vi "Open Handle2.vi"(0 "server address":string caption="サーバアドレス", 5 "from":string caption="送信者", 7 "username":string caption="ユーザ名", 9 "password":string caption="パスワード", 11 "error in (no error)":errorcluster caption="エラー入力（エラーなし）", 12 "use TLS (false)":bool caption="TLSを使用 (FALSE)") -> (4 "handles cluster out":T1 caption="ハンドルクラスター出力", 15 "error out":errorcluster caption="エラー出力")   [LabVIEW 2015]
doc: "指定されたSMTPサーバを使用して新しいハンドルクラスターを作成します。作成したハンドルは、「Close Handle2」VIを使用して閉じる必要があります。"
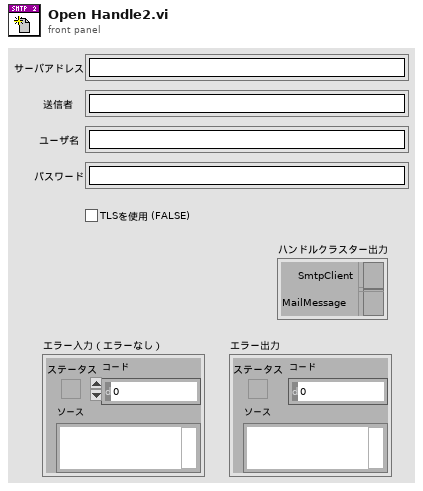
[diagram p1: front panel]
types:
  T1 = cluster{"SmtpClient":refnum<k24>, "MailMessage":refnum<k24>}
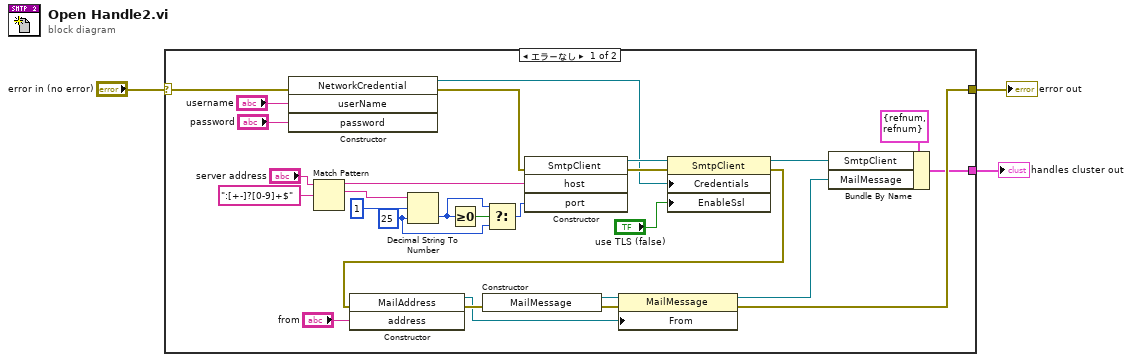
[diagram p0: block diagram]
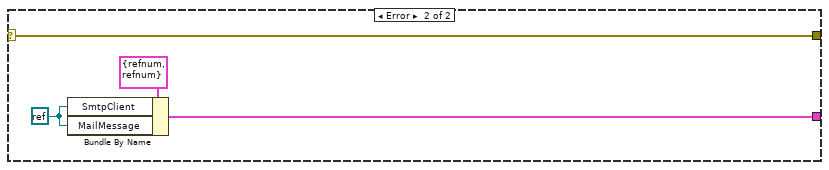
[diagram p2: hidden frame]
diagram:
  n1 = case shown="エラーなし" "error in (no error)" {
    selector: "error in (no error)" -> [w19 w35]
    tunnel: [w5 w35] -> w2
    tunnel: [w4 w32] -> w1
    frame No Error {
      w26 = 25 ("デフォルト（0 I32）")
      n2 = constructor class="NetworkCredential"(error in=w19, "userName"="username", "password"="password") -> (reference out=w16:refnum<k24>, error out=w18:errorcluster)  [unwired: 2 in, 3 out]
      n3 = Match Pattern(string="server address", regular expression=":[+-]?[0-9]+$" ("正規表現")) -> (before substring=w24:string, match substring=w30:string)  [unwired: 1 in, 2 out]
      n4 = Decimal String To Number(string=w30, offset=1 ("オフセット"), default (0L)=w26) -> (number=w27:i32)  [unwired: 1 out]
      n5 = Greater Or Equal To 0?(x=w27) -> (x >= 0?=w28:bool)
      n6 = Select(t=w27, s=w28, f=w26) -> (s? t:f=w17:i32)
      n7 = constructor class="SmtpClient"(error in=w18, "host"=w24, "port"=w17) -> (reference out=w20:refnum<k24>, error out=w21:errorcluster)  [unwired: 2 in, 3 out]
      n8 = property class="SmtpClient"(reference=w20, error in=w21, "Credentials"=w16, "EnableSsl"="use TLS (false)") -> (reference out=w6:refnum<k24>, error out=w10:errorcluster)
      n9 = constructor class="MailAddress"(error in=w10, "address"="from") -> (reference out=w9:refnum<k24>, error out=w14:errorcluster)  [unwired: 2 in, 2 out]
      n10 = constructor class="MailMessage"(error in=w14) -> (reference out=w12:refnum<k24>, error out=w13:errorcluster)  [unwired: 2 in, 1 out]
      n11 = property class="MailMessage"(reference=w12, error in=w13, "From"=w9) -> (reference out=w7:refnum<k24>, error out=w5:errorcluster)
      n12 = Bundle By Name(cluster=T1 {"SmtpClient"=refnum, "MailMessage"=refnum} ("handles cluster out"), "SmtpClient"=w6, "MailMessage"=w7) -> (w4:T1)
    }
    frame Error {
      w33 = refnum<k0> refnum
      n13 = Bundle By Name(cluster=T1 {"SmtpClient"=refnum, "MailMessage"=refnum} ("handles cluster out"), "SmtpClient"=w33, "MailMessage"=w33) -> (w32:T1)
    }
  }
  "handles cluster out" <- w1
  "error out" <- w2
